vi "Get_Active_Port.vi"(8 "error in (no error)":errorcluster, 11 ".NET Reference in":refnum<k24>) -> (0 "error out":errorcluster, 2 "channel":u16, 3 "Reference out":refnum<k24>)   [LabVIEW 2017]
doc: "TSL and OSU optical path check"
uses:
  D:/test/FULLband-sts/Fullband_Sample/DLL/InstrumentDLL.dll
  DLL/InstrumentDLL.dll
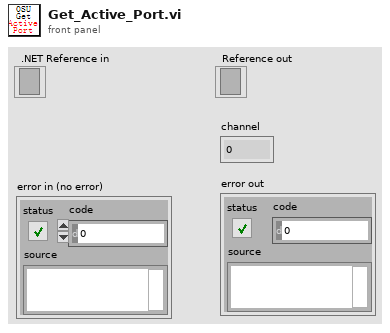
[diagram p1: front panel]
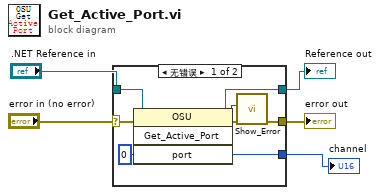
[diagram p0: block diagram]
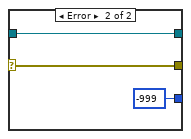
[diagram p2: hidden frame]
diagram:
  n1 = case shown="无错误" "error in (no error)" {
    selector: "error in (no error)" -> [w11 w16]
    tunnel: ".NET Reference in" -> [w13 w15]
    tunnel: [w12 w15] -> w4
    tunnel: [w8 w16] -> w2
    tunnel: [w6 -999 ("port")] -> w1
    frame No Error {
      n2 = invoke on="调用节点" class="OSU" method="Get_Active_Port"(reference=w13, error in=w11, "port"=0) -> (reference out=w12:refnum<k24>, error out=w9:errorcluster, "Get_Active_Port"=w10:i32, "port"=w6:i32)  [unwired: 1 in]
      n3 = call "Show_Error.vi"("error in (no error)"=w9, "Error"=w10) -> ("error out"=w8:errorcluster)  [unwired: 9 in]
    }
    frame Error {
    }
  }
  "channel" <- w1
  "error out" <- w2
  "Reference out" <- w4
